vi "Lab Panel V6.00.vi"() -> ()   [LabVIEW 2017] (continued)
                                n593 = Bundle(cluster=w856, "TL"=w854, "TN"=w854) -> (w855:cluster{"TL":dbl, "TN":dbl})
                                n594 = local write "TEMP START LAB01-1"(w855) -> ()
                              }
                            }
                          }
                        }
                      }
                    }
                  }
                }
              }
              event "RUN LAB01-2": Value Change {
                n595 = event-data() -> ("NewVal"=w861:bool)  [unwired: 1 in, 5 out]
                n596 = local write "run lab01-2"(w861) -> ()
                n597 = case shown="True" w861 {
                  tunnel: w867 -> [_ w905]
                  tunnel: w866 -> [_ w904]
                  tunnel: w864 -> [w869 w903]
                  tunnel: w865 -> [_ w902]
                  tunnel: w863 -> [_ w901]
                  tunnel: [w868 w900] -> w862
                  tunnel: w860 -> [_ w899]
                  tunnel: w859 -> [_ w898]
                  tunnel: w858 -> [_ w897]
                  tunnel: w857 -> [_ w895]
                  frame False {
                    # "stop test"
                    n598 = stacked-sequence {
                      tunnel: w869 -> [w878 _]
                      tunnel: [w870 _] -> w868
                      frame #0 {
                        n599 = local read "DISP LAB01-2"() -> (w877:T4)
                        n600 = Unbundle(w877) -> ("CYCLE"=w875:dbl, "MINS"=w876:dbl)  [unwired: 1 out]
                        n601 = case shown="\"CHART TEST\", Default" w878 {
                          tunnel: w876 -> [_ _ w885]
                          tunnel: w875 -> [w883 w884 _]
                          tunnel: [w883 w884 w885] -> w874
                          frame "CHART TEST", Default {
                          }
                          frame "CYCLE TEST" {
                          }
                          frame "T-RISE TEST" {
                          }
                        }
                        n602 = local read "TDMS LAB01-2"() -> (w882:refnum<k34>)
                        n603 = Build Array("STOPPED") -> (w879:string[])
                        n604 = Build Array(w874) -> (w873:dbl[])
                        n605 = TDMS Write(0:w882, 5:"TEST RESULT", 7:w879, 9:w873) -> (4:w871:refnum<k34>, 15:w872:errorcluster)  [unwired: 2 in, 2 out]
                        n606 = TDMS Close(8:w872, 11:w871) -> (0:w870:errorcluster)  [unwired: 1 out]
                      }
                      frame #1 {
                        n607 = local read "DISP LAB01-2"() -> (w889:T4)
                        n608 = stacked-sequence {
                          tunnel: "LAB01-2" -> [w891 w893]
                          frame #0 {
                            n609 = call "sub vi - defrag tdms v1.vi"("panel id"=w891) -> ("error out"=w890:errorcluster)  [unwired: 10 in]
                            n610 = local write "data file error"(w890) -> ()
                          }
                          frame #1 {
                            n611 = call "Save data file (stop) v3.vi"("panel id"=w893) -> ("network file save error"=w892:errorcluster)  [unwired: 9 in, 1 out]
                            n612 = local write "RESULT LAB01-2"(FALSE) -> ()
                            n613 = local write "data file error"(w892) -> ()
                          }
                        }
                        n614 = Bundle(cluster=w889, "STATUS"="STOP") -> (w887:T4)  [unwired: 2 in]
                        n615 = local write "DISP LAB01-2"(w887) -> ()
                      }
                    }
                  }
                  frame True {
                    n616 = local read "SIG LAB01-2"() -> (w896:T2)
                    n617 = stacked-sequence {
                      seq-local: [w907 _] -> [_ w911]
                      tunnel: w905 -> [_ w921]
                      tunnel: w904 -> [_ w920]
                      tunnel: w903 -> [_ w919]
                      tunnel: w902 -> [_ w918]
                      tunnel: w901 -> [_ w917]
                      tunnel: [_ w916] -> w900
                      tunnel: w899 -> [_ w915]
                      tunnel: w898 -> [_ w914]
                      tunnel: w897 -> [_ w913]
                      tunnel: w896 -> [w906 w912]
                      tunnel: w895 -> [_ w910]
                      frame #0 {
                        n618 = Unbundle(w906) -> ("AMPS"=w909:dbl)  [unwired: 4 out]
                        n619 = call "Check For Amps on v1.vi"("ID"="LAB01-2", "amps"=w909) -> ("amps"=w907:bool)  [unwired: 9 in]
                      }
                      frame #1 {
                        n620 = case shown="True" w911 {
                          tunnel: w921 -> [_ w934]
                          tunnel: w920 -> [_ w933]
                          tunnel: w919 -> [_ w932]
                          tunnel: w918 -> [_ w931]
                          tunnel: w917 -> [_ w930]
                          tunnel: [errorcluster {"status"=FALSE, "code"=0, "source"=""} ("error out") w929] -> w916
                          tunnel: w915 -> [_ w928]
                          tunnel: w914 -> [_ w927]
                          tunnel: w913 -> [_ w926]
                          tunnel: w912 -> [_ w925]
                          tunnel: w910 -> [_ w924]
                          frame False {
                            w922 = FALSE
                            n621 = local write "RUN LAB01-2"(w922) -> ()
                            n622 = local write "run lab01-2"(w922) -> ()
                          }
                          frame True {
                            n623 = stacked-sequence {
                              seq-local: [w935 _ _ _ _] -> [_ w959 _ _ _]
                              tunnel: w934 -> [w940 _ _ _ _]
                              tunnel: w933 -> [w937 _ _ _ _]
                              tunnel: w932 -> [w950 _ _ _ _]
                              tunnel: w931 -> [w943 _ _ _ _]
                              tunnel: w930 -> [w938 _ _ _ _]
                              tunnel: [_ w954 _ _ _] -> w929
                              tunnel: w928 -> [_ _ _ w981 _]
                              tunnel: w927 -> [_ _ _ w980 _]
                              tunnel: w926 -> [_ _ _ w979 _]
                              tunnel: w925 -> [_ _ _ _ _]
                              tunnel: w924 -> [_ _ _ _ w994]
                              frame #0 {
                                w936 = "\\"
                                n624 = local read "SET LAB01-2"() -> (w945:T5)
                                n625 = case shown="\"CYCLE TEST\"" w950 {
                                tunnel: ["L01-2-CHART TEST-" "L01-2-CYCLE TEST-" "L01-2-T-RISE TEST-"] -> w946
                                frame "CHART TEST", Default {
                                }
                                frame "CYCLE TEST" {
                                }
                                frame "T-RISE TEST" {
                                }
                                }
                                n626 = Unbundle(w945) -> ("DESCRIPTION"=w944:string)  [unwired: 4 out]
                                n627 = Concatenate Strings(w940, "\\", w938, w936, w937, w936) -> (w947:string)
                                n628 = String To Path(string=w947) -> (path=w949:path)
                                n629 = Concatenate Strings(w947, w946, w944, "-", w943, ".tdms") -> (w935:string)
                                n630 = Create Folder(path (use dialog)=w949) -> (error out=w948:errorcluster)  [unwired: 2 in, 2 out]
                                n631 = call <vilib>:"Clear Errors.vi"("error in (no error)"=w948) -> ()  [unwired: 5 in, 2 out]
                                n632 = global write "Global 1.vi" "LAB01-2 FILE"(w935) -> ()
                              }
                              frame #1 {
                                (unwired) FALSE
                                n633 = String To Path(string=w959) -> (path=w955:path)
                                n634 = TDMS Open(6:FALSE, 10:T22."create or replace" ("operation (0:open)"), 11:w955) -> (0:w954:errorcluster, 3:→"TDMS LAB01-2":refnum<k34>)  [unwired: 4 in]
                              }
                              frame #2 {
                                n635 = local read "SET LAB01-2"() -> (w965:T5)
                                n636 = local read "TDMS LAB01-2"() -> (w976:refnum<k34>)
                                n637 = Build Array("Testers Name", "Description", "Set Test Cycles", "T-Rise minutes", "T-Rise Deg C") -> (w966:string[])
                                n638 = Unbundle(w965) -> ("NAME"=w964:string, "DESCRIPTION"=w963:string, "CYCLES"=w962:dbl, "T-RISE mins"=w961:dbl, "T-RISE deg C"=w960:dbl)
                                n639 = Number To Decimal String(number=w962) -> (decimal integer string=w975:string)  [unwired: 1 in]
                                n640 = Number To Decimal String(number=w961) -> (decimal integer string=w974:string)  [unwired: 1 in]
                                n641 = Number To Decimal String(number=w960) -> (decimal integer string=w973:string)  [unwired: 1 in]
                                n642 = Build Array(w964, w963, w975, w974, w973) -> (w972:string[])
                                n643 = TDMS Set Properties(5:w972, 7:w966, 11:w976) -> ()  [unwired: 3 in, 4 out]
                              }
                              frame #3 {
                                n644 = local read "DISP LAB01-2"() -> (w978:T4)
                                n645 = Concatenate Strings("LAB01-2  ", w981) -> (w982:string)
                                n646 = Two Button Dialog(message=w982, 1:w979, 2:w980) -> (T button?=w984:bool)
                                n647 = case shown="True" w984 {
                                tunnel: w978 -> [w991 w992]
                                tunnel: [w991 w992] -> w988
                                tunnel: [w990 w993] -> w987
                                tunnel: [w989 w993] -> w986
                                frame False {
                                n648 = Unbundle(w991) -> ("CYCLE"=w990:dbl, "MINS"=w989:dbl)  [unwired: 1 out]
                                }
                                frame True {
                                w993 = 0.0
                                }
                                }
                                n649 = Bundle(cluster=w988, "CYCLE"=w987, "MINS"=w986, "STATUS"="RUN") -> (w977:T4)
                                n650 = local write "DISP LAB01-2"(w977) -> ()
                              }
                              frame #4 {
                                n651 = local read "TEMP START LAB01-2"() -> (w996:cluster{"TL":dbl, "TN":dbl})
                                n652 = Bundle(cluster=w996, "TL"=w994, "TN"=w994) -> (w995:cluster{"TL":dbl, "TN":dbl})
                                n653 = local write "TEMP START LAB01-2"(w995) -> ()
                              }
                            }
                          }
                        }
                      }
                    }
                  }
                }
              }
              event "RUN LAB02-1": Value Change {
                n654 = event-data() -> ("NewVal"=w1002:bool)  [unwired: 1 in, 5 out]
                n655 = local read "SIG LAB02-1"() -> (w998:T2)
                n656 = case shown="True" w1002 {
                  tunnel: w1008 -> [_ w1046]
                  tunnel: w1007 -> [_ w1045]
                  tunnel: w1005 -> [w1010 w1044]
                  tunnel: w1006 -> [_ w1043]
                  tunnel: w1004 -> [_ w1042]
                  tunnel: [w1009 w1041] -> w1003
                  tunnel: w1001 -> [_ w1040]
                  tunnel: w1000 -> [_ w1039]
                  tunnel: w999 -> [_ w1038]
                  tunnel: w998 -> [_ w1037]
                  tunnel: w997 -> [_ w1036]
                  frame False {
                    # "stop test"
                    n657 = stacked-sequence {
                      tunnel: w1010 -> [w1019 _]
                      tunnel: [w1011 _] -> w1009
                      frame #0 {
                        n658 = local read "DISP LAB02-1"() -> (w1018:T4)
                        n659 = Unbundle(w1018) -> ("CYCLE"=w1016:dbl, "MINS"=w1017:dbl)  [unwired: 1 out]
                        n660 = case shown="\"CYCLE TEST\"" w1019 {
                          tunnel: w1017 -> [_ _ w1026]
                          tunnel: w1016 -> [w1024 w1025 _]
                          tunnel: [w1024 w1025 w1026] -> w1015
                          frame "CHART TEST", Default {
                          }
                          frame "CYCLE TEST" {
                          }
                          frame "T-RISE TEST" {
                          }
                        }
                        n661 = local read "TDMS LAB02-1"() -> (w1023:refnum<k34>)
                        n662 = Build Array("STOPPED") -> (w1020:string[])
                        n663 = Build Array(w1015) -> (w1014:dbl[])
                        n664 = TDMS Write(0:w1023, 5:"TEST RESULT", 7:w1020, 9:w1014) -> (4:w1012:refnum<k34>, 15:w1013:errorcluster)  [unwired: 2 in, 2 out]
                        n665 = TDMS Close(8:w1013, 11:w1012) -> (0:w1011:errorcluster)  [unwired: 1 out]
                      }
                      frame #1 {
                        n666 = local read "DISP LAB02-1"() -> (w1030:T4)
                        n667 = stacked-sequence {
                          tunnel: "LAB02-1" -> [w1032 w1034]
                          frame #0 {
                            n668 = call "sub vi - defrag tdms v1.vi"("panel id"=w1032) -> ("error out"=w1031:errorcluster)  [unwired: 10 in]
                            n669 = local write "data file error"(w1031) -> ()
                          }
                          frame #1 {
                            n670 = local write "RESULT LAB02-1"(FALSE) -> ()
                            n671 = call "Save data file (stop) v3.vi"("panel id"=w1034) -> ("network file save error"=w1033:errorcluster)  [unwired: 9 in, 1 out]
                            n672 = local write "data file error"(w1033) -> ()
                          }
                        }
                        n673 = Bundle(cluster=w1030, "STATUS"="STOP") -> (w1028:T4)  [unwired: 2 in]
                        n674 = local write "DISP LAB02-1"(w1028) -> ()
                      }
                    }
                  }
                  frame True {
                    n675 = stacked-sequence {
                      seq-local: [w1048 _] -> [_ w1052]
                      tunnel: w1046 -> [_ w1062]
                      tunnel: w1045 -> [_ w1061]
                      tunnel: w1044 -> [_ w1060]
                      tunnel: w1043 -> [_ w1059]
                      tunnel: w1042 -> [_ w1058]
                      tunnel: [_ w1057] -> w1041
                      tunnel: w1040 -> [_ w1056]
                      tunnel: w1039 -> [_ w1055]
                      tunnel: w1038 -> [_ w1054]
                      tunnel: w1037 -> [w1047 w1053]
                      tunnel: w1036 -> [_ w1051]
                      frame #0 {
                        n676 = Unbundle(w1047) -> ("AMPS"=w1050:dbl)  [unwired: 4 out]
                        n677 = call "Check For Amps on v1.vi"("ID"="LAB02-1", "amps"=w1050) -> ("amps"=w1048:bool)  [unwired: 9 in]
                      }
                      frame #1 {
                        n678 = case shown="True" w1052 {
                          tunnel: w1062 -> [_ w1075]
                          tunnel: w1061 -> [_ w1074]
                          tunnel: w1060 -> [_ w1073]
                          tunnel: w1059 -> [_ w1072]
                          tunnel: w1058 -> [_ w1071]
                          tunnel: [errorcluster {"status"=FALSE, "code"=0, "source"=""} ("error out") w1070] -> w1057
                          tunnel: w1056 -> [_ w1069]
                          tunnel: w1055 -> [_ w1068]
                          tunnel: w1054 -> [_ w1067]
                          tunnel: w1053 -> [_ w1066]
                          tunnel: w1051 -> [_ w1065]
                          frame False {
                            w1064 = FALSE
                            n679 = local write "RUN LAB02-1"(w1064) -> ()
                            n680 = local write "run lab02-1"(w1064) -> ()
                          }
                          frame True {
                            n681 = stacked-sequence {
                              seq-local: [w1076 _ _ _ _] -> [_ w1100 _ _ _]
                              tunnel: w1075 -> [w1081 _ _ _ _]
                              tunnel: w1074 -> [w1078 _ _ _ _]
                              tunnel: w1073 -> [w1091 _ _ _ _]
                              tunnel: w1072 -> [w1084 _ _ _ _]
                              tunnel: w1071 -> [w1079 _ _ _ _]
                              tunnel: [_ w1095 _ _ _] -> w1070
                              tunnel: w1069 -> [_ _ _ w1121 _]
                              tunnel: w1068 -> [_ _ _ w1120 _]
                              tunnel: w1067 -> [_ _ _ w1119 _]
                              tunnel: w1066 -> [_ _ _ _ _]
                              tunnel: w1065 -> [_ _ _ _ w1135]
                              frame #0 {
                                w1077 = "\\"
                                n682 = local read "SET LAB02-1"() -> (w1086:T5)
                                n683 = case shown="\"CYCLE TEST\"" w1091 {
                                tunnel: ["L02-1-CHART TEST-" "L02-1-CYCLE TEST-" "L02-1-T-RISE TEST-"] -> w1087
                                frame "CHART TEST", Default {
                                }
                                frame "CYCLE TEST" {
                                }
                                frame "T-RISE TEST" {
                                }
                                }
                                n684 = Unbundle(w1086) -> ("DESCRIPTION"=w1085:string)  [unwired: 4 out]
                                n685 = Concatenate Strings(w1081, "\\", w1079, w1077, w1078, w1077) -> (w1088:string)
                                n686 = String To Path(string=w1088) -> (path=w1090:path)
                                n687 = Concatenate Strings(w1088, w1087, w1085, "-", w1084, ".tdms") -> (w1076:string)
                                n688 = Create Folder(path (use dialog)=w1090) -> (error out=w1089:errorcluster)  [unwired: 2 in, 2 out]
                                n689 = global write "Global 1.vi" "LAB02-1 FILE"(w1076) -> ()
                                n690 = call <vilib>:"Clear Errors.vi"("error in (no error)"=w1089) -> ()  [unwired: 5 in, 2 out]
                              }
                              frame #1 {
                                (unwired) FALSE
                                n691 = String To Path(string=w1100) -> (path=w1096:path)
                                n692 = TDMS Open(6:FALSE, 10:T22."create or replace" ("operation (0:open)"), 11:w1096) -> (0:w1095:errorcluster, 3:→"TDMS LAB02-1":refnum<k34>)  [unwired: 4 in]
                              }
                              frame #2 {
                                n693 = local read "SET LAB02-1"() -> (w1106:T5)
                                n694 = local read "TDMS LAB02-1"() -> (w1117:refnum<k34>)
                                n695 = Build Array("Testers Name", "Description", "Set Test Cycles", "T-Rise minutes", "T-Rise Deg C") -> (w1107:string[])
                                n696 = Unbundle(w1106) -> ("NAME"=w1105:string, "DESCRIPTION"=w1104:string, "CYCLES"=w1103:dbl, "T-RISE mins"=w1102:dbl, "T-RISE deg C"=w1101:dbl)
                                n697 = Number To Decimal String(number=w1103) -> (decimal integer string=w1116:string)  [unwired: 1 in]
                                n698 = Number To Decimal String(number=w1102) -> (decimal integer string=w1115:string)  [unwired: 1 in]
                                n699 = Number To Decimal String(number=w1101) -> (decimal integer string=w1114:string)  [unwired: 1 in]
                                n700 = Build Array(w1105, w1104, w1116, w1115, w1114) -> (w1113:string[])
                                n701 = TDMS Set Properties(5:w1113, 7:w1107, 11:w1117) -> ()  [unwired: 3 in, 4 out]
                              }
                              frame #3 {
                                n702 = local read "DISP LAB02-1"() -> (w1122:T4)
                                n703 = Concatenate Strings("LAB02-1  ", w1121) -> (w1123:string)
                                n704 = Two Button Dialog(message=w1123, 1:w1119, 2:w1120) -> (T button?=w1125:bool)
                                n705 = case shown="True" w1125 {
                                tunnel: w1122 -> [w1132 w1133]
                                tunnel: [w1132 w1133] -> w1129
                                tunnel: [w1131 w1134] -> w1128
                                tunnel: [w1130 w1134] -> w1127
                                frame False {
                                n706 = Unbundle(w1132) -> ("CYCLE"=w1131:dbl, "MINS"=w1130:dbl)  [unwired: 1 out]
                                }
                                frame True {
                                w1134 = 0.0
                                }
                                }
                                n707 = Bundle(cluster=w1129, "CYCLE"=w1128, "MINS"=w1127, "STATUS"="RUN") -> (w1118:T4)
                                n708 = local write "DISP LAB02-1"(w1118) -> ()
                              }
                              frame #4 {
                                n709 = local read "TEMP START LAB02-1"() -> (w1137:cluster{"TL":dbl, "TN":dbl})
                                n710 = Bundle(cluster=w1137, "TL"=w1135, "TN"=w1135) -> (w1136:cluster{"TL":dbl, "TN":dbl})
                                n711 = local write "TEMP START LAB02-1"(w1136) -> ()
                              }
                            }
                          }
                        }
                      }
                    }
                  }
                }
                n712 = local write "run lab02-1"(w1002) -> ()
              }
              event "RUN LAB02-2": Value Change {
                n713 = event-data() -> ("NewVal"=w1142:bool)  [unwired: 1 in, 5 out]
                n714 = local write "run lab02-2"(w1142) -> ()
                n715 = case shown="True" w1142 {
                  tunnel: w1148 -> [_ w1186]
                  tunnel: w1147 -> [_ w1185]
                  tunnel: w1145 -> [w1150 w1184]
                  tunnel: w1146 -> [_ w1183]
                  tunnel: w1144 -> [_ w1182]
                  tunnel: [w1149 w1181] -> w1143
                  tunnel: w1141 -> [_ w1180]
                  tunnel: w1140 -> [_ w1179]
                  tunnel: w1139 -> [_ w1178]
                  tunnel: w1138 -> [_ w1176]
                  frame False {
                    # "stop test"
                    n716 = stacked-sequence {
                      tunnel: w1150 -> [w1159 _]
                      tunnel: [w1151 _] -> w1149
                      frame #0 {
                        n717 = local read "DISP LAB02-2"() -> (w1158:T4)
                        n718 = Unbundle(w1158) -> ("CYCLE"=w1156:dbl, "MINS"=w1157:dbl)  [unwired: 1 out]
                        n719 = case shown="\"CYCLE TEST\"" w1159 {
                          tunnel: w1157 -> [_ _ w1166]
                          tunnel: w1156 -> [w1164 w1165 _]
                          tunnel: [w1164 w1165 w1166] -> w1155
                          frame "CHART TEST", Default {
                          }
                          frame "CYCLE TEST" {
                          }
                          frame "T-RISE TEST" {
                          }
                        }
                        n720 = local read "TDMS LAB02-2"() -> (w1163:refnum<k34>)
                        n721 = Build Array("STOPPED") -> (w1160:string[])
                        n722 = Build Array(w1155) -> (w1154:dbl[])
                        n723 = TDMS Write(0:w1163, 5:"TEST RESULT", 7:w1160, 9:w1154) -> (4:w1152:refnum<k34>, 15:w1153:errorcluster)  [unwired: 2 in, 2 out]
                        n724 = TDMS Close(8:w1153, 11:w1152) -> (0:w1151:errorcluster)  [unwired: 1 out]
                      }
                      frame #1 {
                        n725 = local read "DISP LAB02-2"() -> (w1170:T4)
                        n726 = stacked-sequence {
                          tunnel: "LAB02-2" -> [w1172 w1174]
                          frame #0 {
                            n727 = call "sub vi - defrag tdms v1.vi"("panel id"=w1172) -> ("error out"=w1171:errorcluster)  [unwired: 10 in]
                            n728 = local write "data file error"(w1171) -> ()
                          }
                          frame #1 {
                            n729 = call "Save data file (stop) v3.vi"("panel id"=w1174) -> ("network file save error"=w1173:errorcluster)  [unwired: 9 in, 1 out]
                            n730 = local write "RESULT LAB02-2"(FALSE) -> ()
                            n731 = local write "data file error"(w1173) -> ()
                          }
                        }
                        n732 = Bundle(cluster=w1170, "STATUS"="STOP") -> (w1168:T4)  [unwired: 2 in]
                        n733 = local write "DISP LAB02-2"(w1168) -> ()
                      }
                    }
                  }
                  frame True {
                    n734 = local read "SIG LAB02-2"() -> (w1177:T2)
                    n735 = stacked-sequence {
                      seq-local: [w1188 _] -> [_ w1192]
                      tunnel: w1186 -> [_ w1202]
                      tunnel: w1185 -> [_ w1201]
                      tunnel: w1184 -> [_ w1200]
                      tunnel: w1183 -> [_ w1199]
                      tunnel: w1182 -> [_ w1198]
                      tunnel: [_ w1197] -> w1181
                      tunnel: w1180 -> [_ w1196]
                      tunnel: w1179 -> [_ w1195]
                      tunnel: w1178 -> [_ w1194]
                      tunnel: w1177 -> [w1187 w1193]
                      tunnel: w1176 -> [_ w1191]
                      frame #0 {
                        n736 = Unbundle(w1187) -> ("AMPS"=w1190:dbl)  [unwired: 4 out]
                        n737 = call "Check For Amps on v1.vi"("ID"="LAB02-2", "amps"=w1190) -> ("amps"=w1188:bool)  [unwired: 9 in]
                      }
                      frame #1 {
                        n738 = case shown="True" w1192 {
                          tunnel: w1202 -> [_ w1215]
                          tunnel: w1201 -> [_ w1214]
                          tunnel: w1200 -> [_ w1213]
                          tunnel: w1199 -> [_ w1212]
                          tunnel: w1198 -> [_ w1211]
                          tunnel: [errorcluster {"status"=FALSE, "code"=0, "source"=""} ("error out") w1210] -> w1197
                          tunnel: w1196 -> [_ w1209]
                          tunnel: w1195 -> [_ w1208]
                          tunnel: w1194 -> [_ w1207]
                          tunnel: w1193 -> [_ w1206]
                          tunnel: w1191 -> [_ w1205]
                          frame False {
                            w1203 = FALSE
                            n739 = local write "RUN LAB02-2"(w1203) -> ()
                            n740 = local write "run lab02-2"(w1203) -> ()
                          }
                          frame True {
                            n741 = stacked-sequence {
                              seq-local: [w1216 _ _ _ _] -> [_ w1240 _ _ _]
                              tunnel: w1215 -> [w1221 _ _ _ _]
                              tunnel: w1214 -> [w1218 _ _ _ _]
                              tunnel: w1213 -> [w1231 _ _ _ _]
                              tunnel: w1212 -> [w1224 _ _ _ _]
                              tunnel: w1211 -> [w1219 _ _ _ _]
                              tunnel: [_ w1235 _ _ _] -> w1210
                              tunnel: w1209 -> [_ _ _ w1261 _]
                              tunnel: w1208 -> [_ _ _ w1260 _]
                              tunnel: w1207 -> [_ _ _ w1259 _]
                              tunnel: w1206 -> [_ _ _ _ _]
                              tunnel: w1205 -> [_ _ _ _ w1275]
                              frame #0 {
                                w1217 = "\\"
                                n742 = local read "SET LAB02-2"() -> (w1226:T5)
                                n743 = case shown="\"CYCLE TEST\"" w1231 {
                                tunnel: ["L02-2-CHART TEST-" "L02-2-CYCLE TEST-" "L02-2-T-RISE TEST-"] -> w1227
                                frame "CHART TEST", Default {
                                }
                                frame "CYCLE TEST" {
                                }
                                frame "T-RISE TEST" {
                                }
                                }
                                n744 = Unbundle(w1226) -> ("DESCRIPTION"=w1225:string)  [unwired: 4 out]
                                n745 = Concatenate Strings(w1221, "\\", w1219, w1217, w1218, w1217) -> (w1228:string)
                                n746 = String To Path(string=w1228) -> (path=w1230:path)
                                n747 = Concatenate Strings(w1228, w1227, w1225, "-", w1224, ".tdms") -> (w1216:string)
                                n748 = Create Folder(path (use dialog)=w1230) -> (error out=w1229:errorcluster)  [unwired: 2 in, 2 out]
                                n749 = global write "Global 1.vi" "LAB02-2 FILE"(w1216) -> ()
                                n750 = call <vilib>:"Clear Errors.vi"("error in (no error)"=w1229) -> ()  [unwired: 5 in, 2 out]
                              }
                              frame #1 {
                                (unwired) FALSE
                                n751 = String To Path(string=w1240) -> (path=w1236:path)
                                n752 = TDMS Open(6:FALSE, 10:T22."create or replace" ("operation (0:open)"), 11:w1236) -> (0:w1235:errorcluster, 3:→"TDMS LAB02-2":refnum<k34>)  [unwired: 4 in]
                              }
                              frame #2 {
                                n753 = local read "SET LAB02-2"() -> (w1246:T5)
                                n754 = local read "TDMS LAB02-2"() -> (w1257:refnum<k34>)
                                n755 = Build Array("Testers Name", "Description", "Set Test Cycles", "T-Rise minutes", "T-Rise Deg C") -> (w1247:string[])
                                n756 = Unbundle(w1246) -> ("NAME"=w1245:string, "DESCRIPTION"=w1244:string, "CYCLES"=w1243:dbl, "T-RISE mins"=w1242:dbl, "T-RISE deg C"=w1241:dbl)
                                n757 = Number To Decimal String(number=w1243) -> (decimal integer string=w1256:string)  [unwired: 1 in]
                                n758 = Number To Decimal String(number=w1242) -> (decimal integer string=w1255:string)  [unwired: 1 in]
                                n759 = Number To Decimal String(number=w1241) -> (decimal integer string=w1254:string)  [unwired: 1 in]
                                n760 = Build Array(w1245, w1244, w1256, w1255, w1254) -> (w1253:string[])
                                n761 = TDMS Set Properties(5:w1253, 7:w1247, 11:w1257) -> ()  [unwired: 3 in, 4 out]
                              }
                              frame #3 {
                                n762 = local read "DISP LAB02-2"() -> (w1262:T4)
                                n763 = Concatenate Strings("LAB02-2  ", w1261) -> (w1263:string)
                                n764 = Two Button Dialog(message=w1263, 1:w1259, 2:w1260) -> (T button?=w1265:bool)
                                n765 = case shown="True" w1265 {
                                tunnel: w1262 -> [w1272 w1273]
                                tunnel: [w1272 w1273] -> w1269
                                tunnel: [w1271 w1274] -> w1268
                                tunnel: [w1270 w1274] -> w1267
                                frame False {
                                n766 = Unbundle(w1272) -> ("CYCLE"=w1271:dbl, "MINS"=w1270:dbl)  [unwired: 1 out]
                                }
                                frame True {
                                w1274 = 0.0
                                }
                                }
                                n767 = Bundle(cluster=w1269, "CYCLE"=w1268, "MINS"=w1267, "STATUS"="RUN") -> (w1258:T4)
                                n768 = local write "DISP LAB02-2"(w1258) -> ()
                              }
                              frame #4 {
                                n769 = local read "TEMP START LAB02-2"() -> (w1277:cluster{"TL":dbl, "TN":dbl})
                                n770 = Bundle(cluster=w1277, "TL"=w1275, "TN"=w1275) -> (w1276:cluster{"TL":dbl, "TN":dbl})
                                n771 = local write "TEMP START LAB02-2"(w1276) -> ()
                              }
                            }
                          }
                        }
                      }
                    }
                  }
                }
              }
              event "RUN LAB03-1": Value Change {
                n772 = event-data() -> ("NewVal"=w1282:bool)  [unwired: 1 in, 5 out]
                n773 = local write "run lab03-1"(w1282) -> ()
                n774 = case shown="True" w1282 {
                  tunnel: w1288 -> [_ w1326]
                  tunnel: w1287 -> [_ w1325]
                  tunnel: w1285 -> [w1290 w1324]
                  tunnel: w1286 -> [_ w1323]
                  tunnel: w1284 -> [_ w1322]
                  tunnel: [w1289 w1321] -> w1283
                  tunnel: w1281 -> [_ w1320]
                  tunnel: w1280 -> [_ w1319]
                  tunnel: w1279 -> [_ w1318]
                  tunnel: w1278 -> [_ w1316]
                  frame False {
                    # "stop test"
                    n775 = stacked-sequence {
                      tunnel: w1290 -> [w1299 _]
                      tunnel: [w1291 _] -> w1289
                      frame #0 {
                        n776 = local read "DISP LAB03-1"() -> (w1298:T4)
                        n777 = Unbundle(w1298) -> ("CYCLE"=w1296:dbl, "MINS"=w1297:dbl)  [unwired: 1 out]
                        n778 = case shown="\"CYCLE TEST\"" w1299 {
                          tunnel: w1297 -> [_ _ w1306]
                          tunnel: w1296 -> [w1304 w1305 _]
                          tunnel: [w1304 w1305 w1306] -> w1295
                          frame "CHART TEST", Default {
                          }
                          frame "CYCLE TEST" {
                          }
                          frame "T-RISE TEST" {
                          }
                        }
                        n779 = local read "TDMS LAB03-1"() -> (w1303:refnum<k34>)
                        n780 = Build Array("STOPPED") -> (w1300:string[])
                        n781 = Build Array(w1295) -> (w1294:dbl[])
                        n782 = TDMS Write(0:w1303, 5:"TEST RESULT", 7:w1300, 9:w1294) -> (4:w1292:refnum<k34>, 15:w1293:errorcluster)  [unwired: 2 in, 2 out]
                        n783 = TDMS Close(8:w1293, 11:w1292) -> (0:w1291:errorcluster)  [unwired: 1 out]
                      }
                      frame #1 {
                        n784 = local read "DISP LAB03-1"() -> (w1310:T4)
                        n785 = stacked-sequence {
                          tunnel: "LAB03-1" -> [w1312 w1314]
                          frame #0 {
                            n786 = call "sub vi - defrag tdms v1.vi"("panel id"=w1312) -> ("error out"=w1311:errorcluster)  [unwired: 10 in]
                            n787 = local write "data file error"(w1311) -> ()
                          }
                          frame #1 {
                            n788 = call "Save data file (stop) v3.vi"("panel id"=w1314) -> ("network file save error"=w1313:errorcluster)  [unwired: 9 in, 1 out]
                            n789 = local write "RESULT LAB03-1"(FALSE) -> ()
                            n790 = local write "data file error"(w1313) -> ()
                          }
                        }
                        n791 = Bundle(cluster=w1310, "STATUS"="STOP") -> (w1308:T4)  [unwired: 2 in]
                        n792 = local write "DISP LAB03-1"(w1308) -> ()
                      }
                    }
                  }
                  frame True {
                    n793 = local read "SIG LAB03-1"() -> (w1317:T2)
                    n794 = stacked-sequence {
                      seq-local: [w1328 _] -> [_ w1332]
                      tunnel: w1326 -> [_ w1342]
                      tunnel: w1325 -> [_ w1341]
                      tunnel: w1324 -> [_ w1340]
                      tunnel: w1323 -> [_ w1339]
                      tunnel: w1322 -> [_ w1338]
                      tunnel: [_ w1337] -> w1321
                      tunnel: w1320 -> [_ w1336]
                      tunnel: w1319 -> [_ w1335]
                      tunnel: w1318 -> [_ w1334]
                      tunnel: w1317 -> [w1327 w1333]
                      tunnel: w1316 -> [_ w1331]
                      frame #0 {
                        n795 = Unbundle(w1327) -> ("AMPS"=w1330:dbl)  [unwired: 4 out]
                        n796 = call "Check For Amps on v1.vi"("ID"="LAB03-1", "amps"=w1330) -> ("amps"=w1328:bool)  [unwired: 9 in]
                      }
                      frame #1 {
                        n797 = case shown="True" w1332 {
                          tunnel: w1342 -> [_ w1355]
                          tunnel: w1341 -> [_ w1354]
                          tunnel: w1340 -> [_ w1353]
                          tunnel: w1339 -> [_ w1352]
                          tunnel: w1338 -> [_ w1351]
                          tunnel: [errorcluster {"status"=FALSE, "code"=0, "source"=""} ("error out") w1350] -> w1337
                          tunnel: w1336 -> [_ w1349]
                          tunnel: w1335 -> [_ w1348]
                          tunnel: w1334 -> [_ w1347]
                          tunnel: w1333 -> [_ w1346]
                          tunnel: w1331 -> [_ w1345]
                          frame False {
                            w1343 = FALSE
                            n798 = local write "RUN LAB03-1"(w1343) -> ()
                            n799 = local write "run lab03-1"(w1343) -> ()
                          }
                          frame True {
                            n800 = stacked-sequence {
                              seq-local: [w1356 _ _ _ _] -> [_ w1380 _ _ _]
                              tunnel: w1355 -> [w1361 _ _ _ _]
                              tunnel: w1354 -> [w1358 _ _ _ _]
                              tunnel: w1353 -> [w1371 _ _ _ _]
                              tunnel: w1352 -> [w1364 _ _ _ _]
                              tunnel: w1351 -> [w1359 _ _ _ _]
                              tunnel: [_ w1375 _ _ _] -> w1350
                              tunnel: w1349 -> [_ _ _ w1400 _]
                              tunnel: w1348 -> [_ _ _ w1399 _]
                              tunnel: w1347 -> [_ _ _ w1398 _]
                              tunnel: w1346 -> [_ _ _ _ _]
                              tunnel: w1345 -> [_ _ _ _ w1415]
                              frame #0 {
                                w1357 = "\\"
                                n801 = local read "SET LAB03-1"() -> (w1366:T5)
                                n802 = case shown="\"T-RISE TEST\"" w1371 {
                                tunnel: ["L03-1-CHART TEST-" "L03-1-CYCLE TEST-" "L03-1-T-RISE TEST-"] -> w1367
                                frame "CHART TEST", Default {
                                }
                                frame "CYCLE TEST" {
                                }
                                frame "T-RISE TEST" {
                                }
                                }
                                n803 = Unbundle(w1366) -> ("DESCRIPTION"=w1365:string)  [unwired: 4 out]
                                n804 = Concatenate Strings(w1361, "\\", w1359, w1357, w1358, w1357) -> (w1368:string)
                                n805 = String To Path(string=w1368) -> (path=w1370:path)
                                n806 = Concatenate Strings(w1368, w1367, w1365, "-", w1364, ".tdms") -> (w1356:string)
                                n807 = Create Folder(path (use dialog)=w1370) -> (error out=w1369:errorcluster)  [unwired: 2 in, 2 out]
                                n808 = global write "Global 1.vi" "LAB03-1 FILE"(w1356) -> ()
                                n809 = call <vilib>:"Clear Errors.vi"("error in (no error)"=w1369) -> ()  [unwired: 5 in, 2 out]
                              }
                              frame #1 {
                                (unwired) FALSE
                                n810 = String To Path(string=w1380) -> (path=w1376:path)
                                n811 = TDMS Open(6:FALSE, 10:T22."create or replace" ("operation (0:open)"), 11:w1376) -> (0:w1375:errorcluster, 3:→"TDMS LAB03-1":refnum<k34>)  [unwired: 4 in]
                              }
                              frame #2 {
                                n812 = local read "SET LAB03-1"() -> (w1386:T5)
                                n813 = local read "TDMS LAB03-1"() -> (w1397:refnum<k34>)
                                n814 = Build Array("Testers Name", "Description", "Set Test Cycles", "T-Rise minutes", "T-Rise Deg C") -> (w1387:string[])
                                n815 = Unbundle(w1386) -> ("NAME"=w1385:string, "DESCRIPTION"=w1384:string, "CYCLES"=w1383:dbl, "T-RISE mins"=w1382:dbl, "T-RISE deg C"=w1381:dbl)
                                n816 = Number To Decimal String(number=w1383) -> (decimal integer string=w1396:string)  [unwired: 1 in]
                                n817 = Number To Decimal String(number=w1382) -> (decimal integer string=w1395:string)  [unwired: 1 in]
                                n818 = Number To Decimal String(number=w1381) -> (decimal integer string=w1394:string)  [unwired: 1 in]
                                n819 = Build Array(w1385, w1384, w1396, w1395, w1394) -> (w1393:string[])
                                n820 = TDMS Set Properties(5:w1393, 7:w1387, 11:w1397) -> ()  [unwired: 3 in, 4 out]
                              }
                              frame #3 {
                                n821 = local read "DISP LAB03-1"() -> (w1402:T4)
                                n822 = Concatenate Strings("LAB03-1  ", w1400) -> (w1403:string)
                                n823 = Two Button Dialog(message=w1403, 1:w1398, 2:w1399) -> (T button?=w1405:bool)
                                n824 = case shown="True" w1405 {
                                tunnel: w1402 -> [w1412 w1413]
                                tunnel: [w1412 w1413] -> w1409
                                tunnel: [w1411 w1414] -> w1408
                                tunnel: [w1410 w1414] -> w1407
                                frame False {
                                n825 = Unbundle(w1412) -> ("CYCLE"=w1411:dbl, "MINS"=w1410:dbl)  [unwired: 1 out]
                                }
                                frame True {
                                w1414 = 0.0
                                }
                                }
                                n826 = Bundle(cluster=w1409, "CYCLE"=w1408, "MINS"=w1407, "STATUS"="RUN") -> (w1401:T4)
                                n827 = local write "DISP LAB03-1"(w1401) -> ()
                              }
                              frame #4 {
                                n828 = local read "TEMP START LAB03-1"() -> (w1417:cluster{"TL":dbl, "TN":dbl})
                                n829 = Bundle(cluster=w1417, "TL"=w1415, "TN"=w1415) -> (w1416:cluster{"TL":dbl, "TN":dbl})
                                n830 = local write "TEMP START LAB03-1"(w1416) -> ()
                              }
                            }
                          }
                        }
                      }
                    }
                  }
                }
              }
              event "RUN LAB03-2": Value Change {
                n831 = event-data() -> ("NewVal"=w1422:bool)  [unwired: 1 in, 5 out]
                n832 = local write "run lab03-2"(w1422) -> ()
                n833 = case shown="True" w1422 {
                  tunnel: w1428 -> [_ w1466]
                  tunnel: w1427 -> [_ w1465]
                  tunnel: w1425 -> [w1430 w1464]
                  tunnel: w1426 -> [_ w1463]
                  tunnel: w1424 -> [_ w1462]
                  tunnel: [w1429 w1461] -> w1423
                  tunnel: w1421 -> [_ w1460]
                  tunnel: w1420 -> [_ w1459]
                  tunnel: w1419 -> [_ w1458]
                  tunnel: w1418 -> [_ w1456]
                  frame False {
                    # "stop test"
                    n834 = stacked-sequence {
                      tunnel: w1430 -> [w1439 _]
                      tunnel: [w1431 _] -> w1429
                      frame #0 {
                        n835 = local read "DISP LAB03-2"() -> (w1438:T4)
                        n836 = Unbundle(w1438) -> ("CYCLE"=w1436:dbl, "MINS"=w1437:dbl)  [unwired: 1 out]
                        n837 = case shown="\"CYCLE TEST\"" w1439 {
                          tunnel: w1437 -> [_ _ w1446]
                          tunnel: w1436 -> [w1444 w1445 _]
                          tunnel: [w1444 w1445 w1446] -> w1435
                          frame "CHART TEST", Default {
                          }
                          frame "CYCLE TEST" {
                          }
                          frame "T-RISE TEST" {
                          }
                        }
                        n838 = local read "TDMS LAB03-2"() -> (w1443:refnum<k34>)
                        n839 = Build Array("STOPPED") -> (w1440:string[])
                        n840 = Build Array(w1435) -> (w1434:dbl[])
                        n841 = TDMS Write(0:w1443, 5:"TEST RESULT", 7:w1440, 9:w1434) -> (4:w1432:refnum<k34>, 15:w1433:errorcluster)  [unwired: 2 in, 2 out]
                        n842 = TDMS Close(8:w1433, 11:w1432) -> (0:w1431:errorcluster)  [unwired: 1 out]
                      }
                      frame #1 {
                        n843 = local read "DISP LAB03-2"() -> (w1450:T4)
                        n844 = stacked-sequence {
                          tunnel: "LAB03-2" -> [w1452 w1454]
                          frame #0 {
                            n845 = call "sub vi - defrag tdms v1.vi"("panel id"=w1452) -> ("error out"=w1451:errorcluster)  [unwired: 10 in]
                            n846 = local write "data file error"(w1451) -> ()
                          }
                          frame #1 {
                            n847 = call "Save data file (stop) v3.vi"("panel id"=w1454) -> ("network file save error"=w1453:errorcluster)  [unwired: 9 in, 1 out]
                            n848 = local write "RESULT LAB03-2"(FALSE) -> ()
                            n849 = local write "data file error"(w1453) -> ()
                          }
                        }
                        n850 = Bundle(cluster=w1450, "STATUS"="STOP") -> (w1448:T4)  [unwired: 2 in]
                        n851 = local write "DISP LAB03-2"(w1448) -> ()
                      }
                    }
                  }
                  frame True {
                    n852 = local read "SIG LAB03-2"() -> (w1457:T2)
                    n853 = stacked-sequence {
                      seq-local: [w1468 _] -> [_ w1472]
                      tunnel: w1466 -> [_ w1482]
                      tunnel: w1465 -> [_ w1481]
                      tunnel: w1464 -> [_ w1480]
                      tunnel: w1463 -> [_ w1479]
                      tunnel: w1462 -> [_ w1478]
                      tunnel: [_ w1477] -> w1461
                      tunnel: w1460 -> [_ w1476]
                      tunnel: w1459 -> [_ w1475]
                      tunnel: w1458 -> [_ w1474]
                      tunnel: w1457 -> [w1467 w1473]
                      tunnel: w1456 -> [_ w1471]
                      frame #0 {
                        n854 = Unbundle(w1467) -> ("AMPS"=w1470:dbl)  [unwired: 4 out]
                        n855 = call "Check For Amps on v1.vi"("ID"="LAB03-2", "amps"=w1470) -> ("amps"=w1468:bool)  [unwired: 9 in]
                      }
                      frame #1 {
                        n856 = case shown="True" w1472 {
                          tunnel: w1482 -> [_ w1495]
                          tunnel: w1481 -> [_ w1494]
                          tunnel: w1480 -> [_ w1493]
                          tunnel: w1479 -> [_ w1492]
                          tunnel: w1478 -> [_ w1491]
                          tunnel: [errorcluster {"status"=FALSE, "code"=0, "source"=""} ("error out") w1490] -> w1477
                          tunnel: w1476 -> [_ w1489]
                          tunnel: w1475 -> [_ w1488]
                          tunnel: w1474 -> [_ w1487]
                          tunnel: w1473 -> [_ w1486]
                          tunnel: w1471 -> [_ w1485]
                          frame False {
                            w1483 = FALSE
                            n857 = local write "RUN LAB03-2"(w1483) -> ()
                            n858 = local write "run lab03-2"(w1483) -> ()
                          }
                          frame True {
                            n859 = stacked-sequence {
                              seq-local: [w1496 _ _ _ _] -> [_ w1520 _ _ _]
                              tunnel: w1495 -> [w1501 _ _ _ _]
                              tunnel: w1494 -> [w1498 _ _ _ _]
                              tunnel: w1493 -> [w1511 _ _ _ _]
                              tunnel: w1492 -> [w1504 _ _ _ _]
                              tunnel: w1491 -> [w1499 _ _ _ _]
                              tunnel: [_ w1515 _ _ _] -> w1490
                              tunnel: w1489 -> [_ _ _ w1541 _]
                              tunnel: w1488 -> [_ _ _ w1540 _]
                              tunnel: w1487 -> [_ _ _ w1539 _]
                              tunnel: w1486 -> [_ _ _ _ _]
                              tunnel: w1485 -> [_ _ _ _ w1555]
                              frame #0 {
                                w1497 = "\\"
